vi "BRig_dataLC_Cue_First_Block_l1.vi"() -> (2 "output_Cue_First_Block":i32)   [LabVIEW 2014]
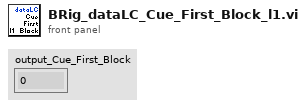
[diagram p1: front panel]
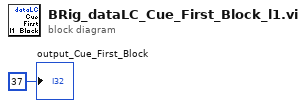
[diagram p0: block diagram]
diagram:
  "output_Cue_First_Block" <- 37 ("output_iBlock")
